vi "Configure Sense Detector.vi"(0 "VISA resource name":refnum<visa-resource-name>, 5 "Sense Source (0: Internal)":u16(ring) items=["Internal", "External"], 7 "Closed Loop Feedback Type (0: Real Time)":u16(ring) items=["Real Time", "RMS"], 11 "error in (no error)":errorcluster) -> (4 "VISA resource name out":refnum<visa-resource-name>, 15 "error out":errorcluster)   [LabVIEW 2020, in "Agilent 681x Series.lvlib"]
doc: "Configures the voltage sensing and closed loop feedback settings."
uses:
  <instrlib>/Agilent 681x Series/Agilent 681x Series.lvlib
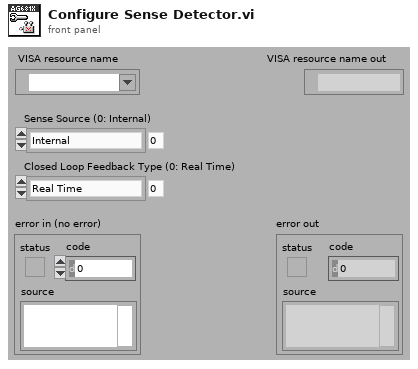
[diagram p1: front panel]
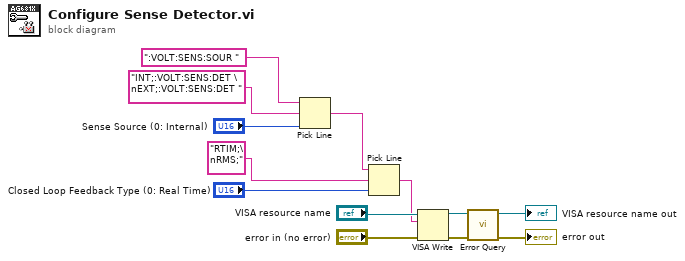
[diagram p0: block diagram]
diagram:
  n1 = Pick Line(string ("")=":VOLT:SENS:SOUR ", multi-line string="INT;:VOLT:SENS:DET \nEXT;:VOLT:SENS:DET ", line index="Sense Source (0: Internal)") -> (output string=w2:string)
  n2 = Pick Line(string ("")=w2, multi-line string="RTIM;\nRMS;", line index="Closed Loop Feedback Type (0: Real Time)") -> (output string=w1:string)
  n3 = VISA Write(VISA resource name="VISA resource name", write buffer=w1, error in (no error)="error in (no error)") -> (VISA resource name out=w11:refnum<visa-resource-name>, error out=w10:errorcluster)  [unwired: 1 out]
  n4 = call <instrlib>:"Error Query.vi"("error in (no error)"=w10, "VISA resource name"=w11) -> ("error out"=→"error out":errorcluster, "VISA resource name out"=→"VISA resource name out":refnum<visa-resource-name>)  [unwired: 6 in, 2 out]
